vi "ZCAN_InitLIN(USBCANFD).vi"(0 "device_hande":u32, 5 "lin_index":u32, 11 "error in (no error)":errorcluster caption="错误输入（无错误）", 13 "ZCAN_LIN_INIT_CONFIG_USBCANFD":T1) -> (8 "LIN_index_handle":u32, 15 "error out":errorcluster caption="错误输出")   [LabVIEW 2020, in "zlgcan.lvlib"]
uses:
  zlgcan.lvlib
  ZCAN_LIN_INIT_CONFIG_USBCANFD.ctl
  bin/zlgcan_wrap.dll
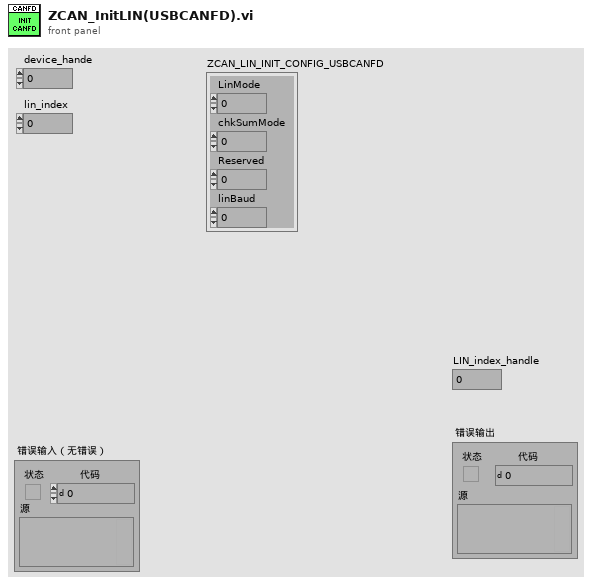
[diagram p1: front panel]
types:
  T1 = typedef "zlgcan.lvlib/ZCAN_LIN_INIT_CONFIG_USBCANFD.ctl" = cluster{"LinMode":u8, "chkSumMode":u8, "Reserved":u16, "linBaud":u32}
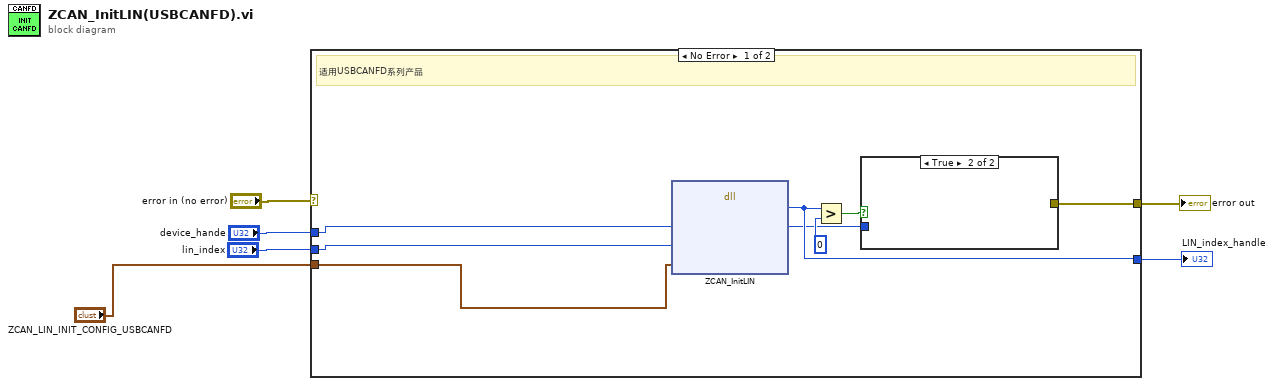
[diagram p0: block diagram]
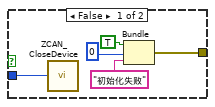
[diagram p2: hidden frame]
diagram:
  n1 = case shown="No Error" "error in (no error)" {
    selector: "error in (no error)" -> [_ w20]
    tunnel: [w14 w20] -> w5
    tunnel: "device_hande" -> [w9 _]
    tunnel: "lin_index" -> [w8 _]
    tunnel: [w13 _] -> w2
    tunnel: "ZCAN_LIN_INIT_CONFIG_USBCANFD" -> [w7 _]
    frame No Error {
      # "适用USBCANFD系列产品"
      n2 = dll-call lib="E:/Jabil tools/JabilTestLib/ZLG_CANFD/bin/zlgcan_wrap.dll" fn="ZCAN_InitLIN" ("ZCAN_InitCAN")("device_handle"=w9, "can_index"=w8, "pInitConfig"=w7) -> ("can_handle"=w13:u32, "device_handle"=w10:u32)  [unwired: 5 in, 2 out]
      n3 = Greater?(x=w13, y=0) -> (0:w11:bool)
      n4 = case shown="True" w11 {
        tunnel: [w16 _] -> w14
        tunnel: w10 -> [w15 _]
        frame False {
          n5 = call "ZCAN_CloseDevice.vi"("device_handle"=w15) -> ()  [unwired: 9 in, 2 out]
          n6 = Bundle("status"=TRUE, "code"=0, "消息"="初始化失败") -> (w16:cluster{"status":bool, "code":i32, "消息":string})  [unwired: 1 in]
        }
        frame True {
        }
      }
    }
    frame Error {
    }
  }
  "error out" <- w5
  "LIN_index_handle" <- w2
